vi "add object (SubVI).vi"(4 "Particle Measurements (Pixels)":dbl[](array[numeric]), 5 "output array in":string[][](array[string]), 6 "Cluster":T1, 7 "contours in":T2(array[cluster]), 8 "metrics":cluster{"Boolean":bool, "String":string}[](array[cluster]), 9 "category":u16, 10 "Picture":i32, 11 "Object in":i32) -> (0 "Array":string[](array[string]), 1 "contours out":T2(array[cluster]), 2 "output array out":string[][](array[string]), 3 "Object out":i32)   [LabVIEW 2020]
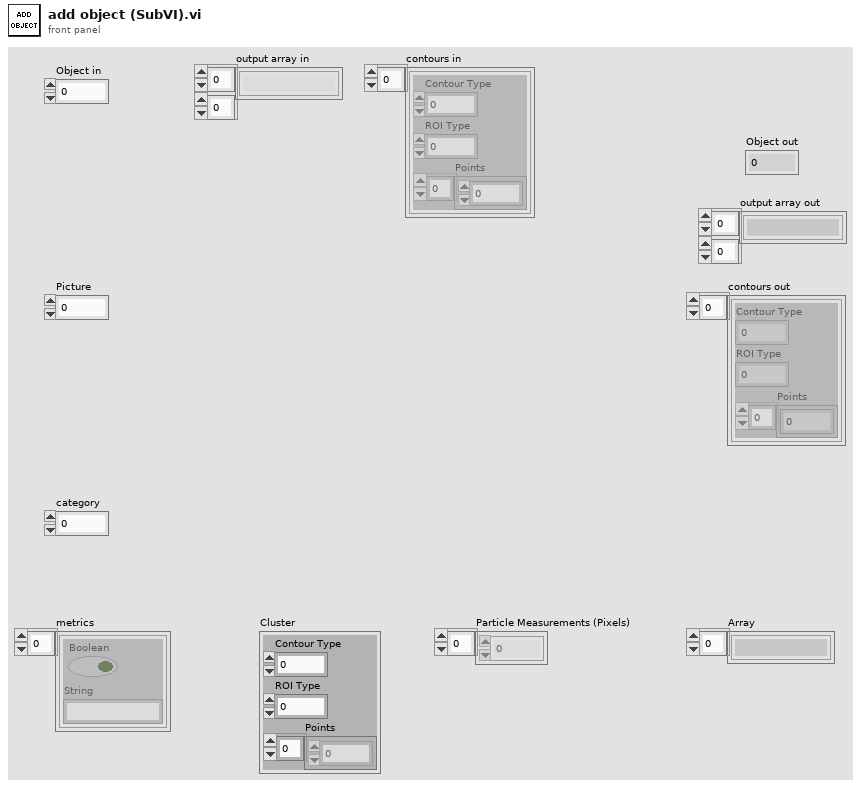
[diagram p1: front panel]
types:
  T1 = cluster{"Contour Type":u32, "ROI Type":u32, "Points":i32[]}
  T2 = cluster{"Contour Type":u32, "ROI Type":u32, "Points":i32[]}[]
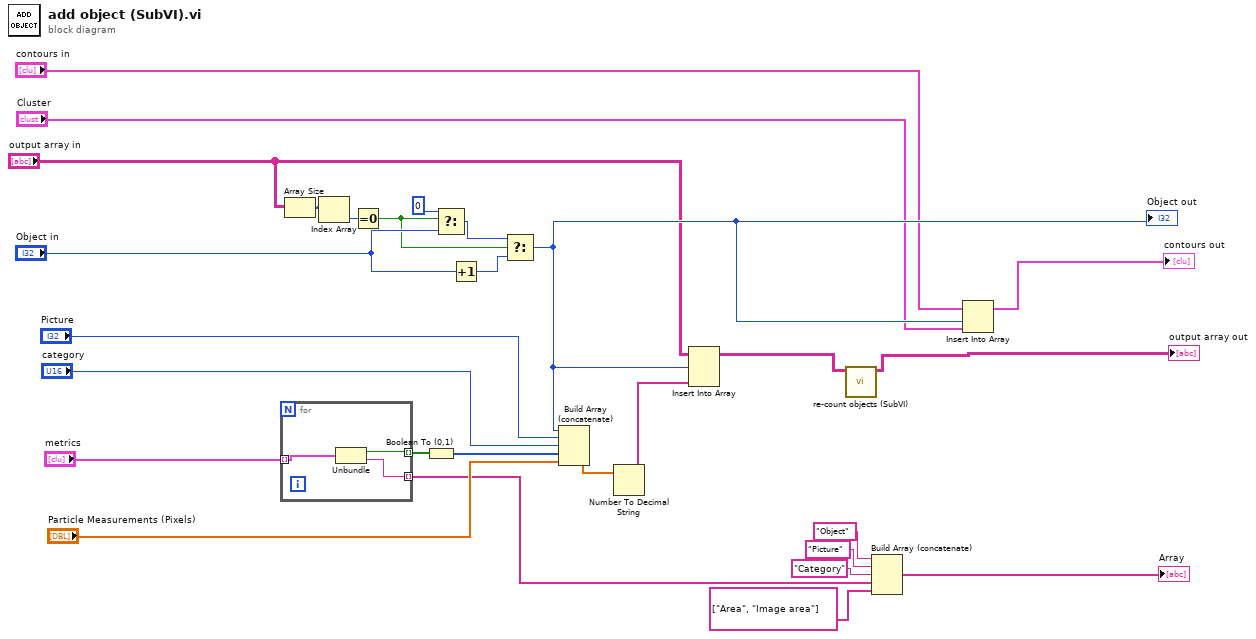
[diagram p0: block diagram]
diagram:
  n1 = for {
    tunnel: "metrics" -> [w31] mode=indexing
    tunnel: [w30] -> w12 mode=indexing
    tunnel: [w29] -> w13 mode=indexing
    n2 = Unbundle(w31) -> ("Boolean"=w30:bool, "String"=w29:string)
  }
  n3 = Array Size(array="output array in") -> (size(s)=w20:i32[])
  n4 = Index Array(array=w20) -> (element=w21:i32)  [unwired: 1 in]
  n5 = Equal To 0?(x=w21) -> (x = 0?=w23:bool)
  n6 = Boolean To (0,1)(Boolean=w12) -> (0, 1=w3:i16[])
  n7 = Select(t=0 ("Object"), s=w23, f="Object in") -> (s? t:f=w25:i32)
  n8 = Increment(x="Object in") -> (x+1=w24:i32)
  n9 = Select(t=w25, s=w23, f=w24) -> (s? t:f=w27:i32)
  "Object out" <- w27
  n10 = Build Array (concatenate)(w27, "Picture", "category", w3, "Particle Measurements (Pixels)") -> (w4:dbl[])
  n11 = Number To Decimal String(number=w4) -> (decimal integer string=w9:string[])  [unwired: 1 in]
  n12 = Insert Into Array(array="output array in", index (row)=w27, new element=w9) -> (w2:string[][])  [unwired: 1 in]
  n13 = call "re-count objects (SubVI).vi"("output array in in"=w2) -> ("output array out"=→"output array out":string[][])  [unwired: 10 in]
  n14 = Build Array (concatenate)("Object" ("element"), "Picture", "Category", w13, string[] ["Area", "Image area"] ("appended array")) -> (→"Array":string[])
  n15 = Insert Into Array(array="contours in", index=w27, new element="Cluster") -> (→"contours out":T2)
